vi "Test_FormatType_EmptyInput_NoErrorOut.vi"(8 "error in (no error)":errorcluster, 11 "TestCase in":refnum<class "TestVariantExtensions.lvclass">) -> (0 "error out":errorcluster, 3 "TestCase out":refnum<class "TestVariantExtensions.lvclass">)   [LabVIEW 2017, in "TestVariantExtensions.lvclass"]
uses:
  TestVariantExtensions.lvclass
  Source/VariantExtensions.lvlib
panel:
  out "Name String":string
  out "Returned Error (None)":errorcluster
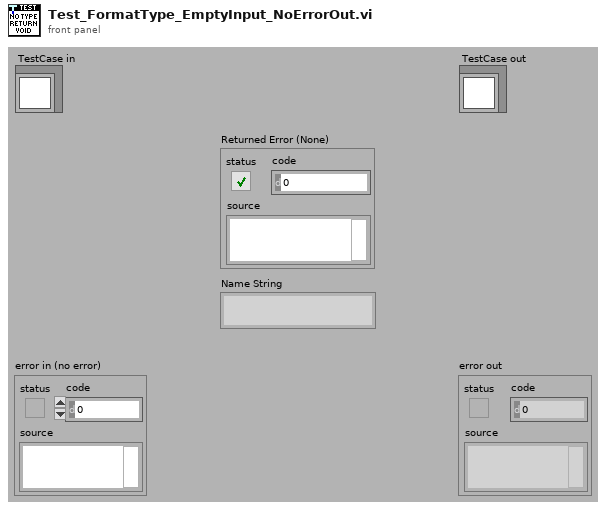
[diagram p1: front panel]
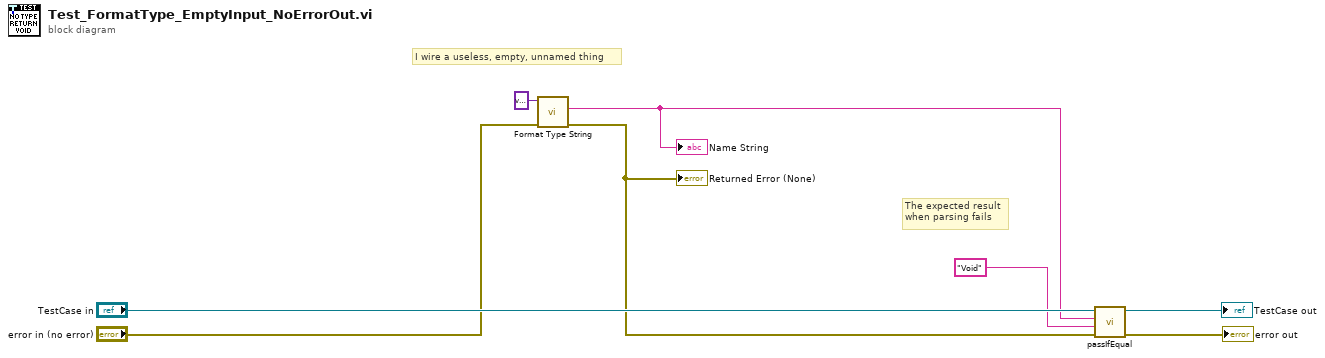
[diagram p0: block diagram]
diagram:
  # "The expected result\nwhen parsing fails"
  # "I wire a useless, empty, unnamed thing"
  n1 = call "Format Type String.vi"("error in (no error)"="error in (no error)", "Data Type"=variant) -> ("error out"=w2:errorcluster, "Type Name"=w5:string)  [unwired: 8 in]
  "Returned Error (None)" <- w2
  "Name String" <- w5
  n2 = call-dynamic "passIfEqual.vi"("error in (no error)"=w2, "y"="Void", "x"=w5, "TestCase in"="TestCase in") -> ("error out"=→"error out":errorcluster, "TestCase out"=→"TestCase out":refnum<class "TestVariantExtensions.lvclass">)  [unwired: 6 in]
